vi "Is Null.vi"(3 "MessageQ in":refnum<class "MessageQ.lvclass">) -> (1 "Null":bool)   [LabVIEW 2020, in "Volatus.lvlib" / "MessageQ.lvclass"]
uses:
  MessageQ.lvclass
  MessageQ.lvclass/MessageQ.ctl
  Message.ctl
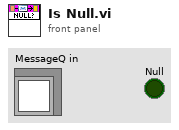
[diagram p1: front panel]
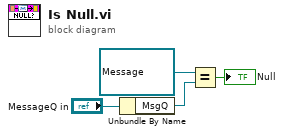
[diagram p0: block diagram]
diagram:
  n1 = Unbundle By Name("MessageQ in") -> ("MsgQ"=w3:refnum<queue>)
  n2 = Equal?(x=refnum<queue> refnum ("y"), y=w3) -> (x = y?=→"Null":bool)
